vi "RPM.vi"(3 "factor":dbl, 4 "Lower level":dbl, 5 "data":dbl) -> (0 "km/h":dbl, 1 "RPM":dbl, 2 "Frequency":dbl)   [LabVIEW 2014]
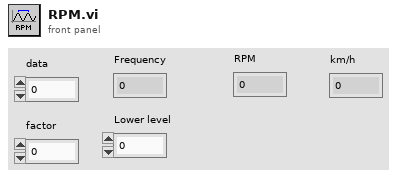
[diagram p1: front panel]
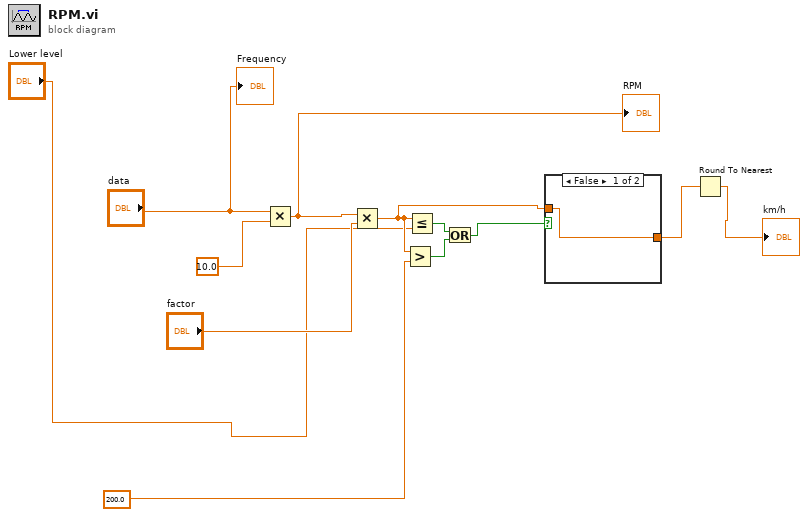
[diagram p0: block diagram]
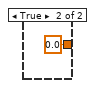
[diagram p2: hidden frame]
diagram:
  n1 = Multiply(x="data", y=10.0) -> (x*y=w4:dbl)
  "RPM" <- w4
  n2 = Multiply(x=w4, y="factor") -> (x*y=w9:dbl)
  n3 = Greater?(x=w9, y=200.0 ("Low Base speed")) -> (0:w8:bool)
  n4 = Less Or Equal?(x=w9, y="Lower level") -> (x <= y?=w7:bool)
  n5 = Or(x=w7, y=w8) -> (x .or. y?=w6:bool)
  n6 = case shown="False" w6 {
    tunnel: [w13 0.0 ("km/h")] -> w3
    tunnel: w9 -> [w13 _]
    frame False {
    }
    frame True {
    }
  }
  n7 = Round To Nearest(number=w3) -> (nearest integer value=→"km/h":dbl)
  "Frequency" <- "data"
